vi "Oscillo2Data.vi"() -> ()   [LabVIEW 2023]
panel:
  out "standard error":string
  out "Extract path 2":path
  out "Current VI folder 2":path
  out "PNG file name 2":string
  out "Traces.txt 2":string
  out "Script.m path 2":path
  out "PDF file path 2":path
  out "Pixmap.bin path 2":path
  out "Traces.txt path 2":path
  in  "User interface":T1(tab)
  in  "User entries":enum32{""}(tab)
  in  "Customization":enum32{"Customization"}(tab)
  in  "Marker shape":string
  in  "Marker size":i32
  in  "Open PDF":bool
  in  "Open in MATLAB":bool
  in  "Colors":enum32{"Colors"}(tab)
  out "Corners":u32(colorbox)
  out "Traces":u32[](array[colorbox])
  in  "Size":enum32{"Size"}(tab)
  out "Depth":i32
  out "Width":i16
  out "Height":i16
  out "stdout":string
  in  "PNG file path":path
  out "Errors":string
  out "PNG picture":picture
  out "Current VI folder":path
  out "PNG file name":string
  out "Pixmap.bin path":path
  out "Traces.txt path":path
  out "Extract path":path
  out "Script.m path":path
  out "PDF file path":path
  out "Traces.txt":string
  in  "Arrays":enum32{"Arrays"}(tab)
  out "Pixels colors (uchar)":u32[](array[numeric])
  out "Pixels colors (CLUT)":u8[](array[numeric])
  out "Corners color (CLUT)":i32
  out "Traces colors (RGB)":u8[][](array[numeric])
  out "Traces colors (CLUT)":i32[](array[numeric])
  out "Traces colors string (RGB)":string[](array[string])
  out "Number of Traces":i32
  out "Script.m":string
  out "Colors error":errorcluster
  out "PNGFile error":errorcluster
  out "PixmapWrite error":errorcluster
  out "CallExtract error":errorcluster
  out "CallMATLAB out":errorcluster
  out "ScriptWrite error":errorcluster
  out "TracesRead error":errorcluster
  out "Paths error":errorcluster
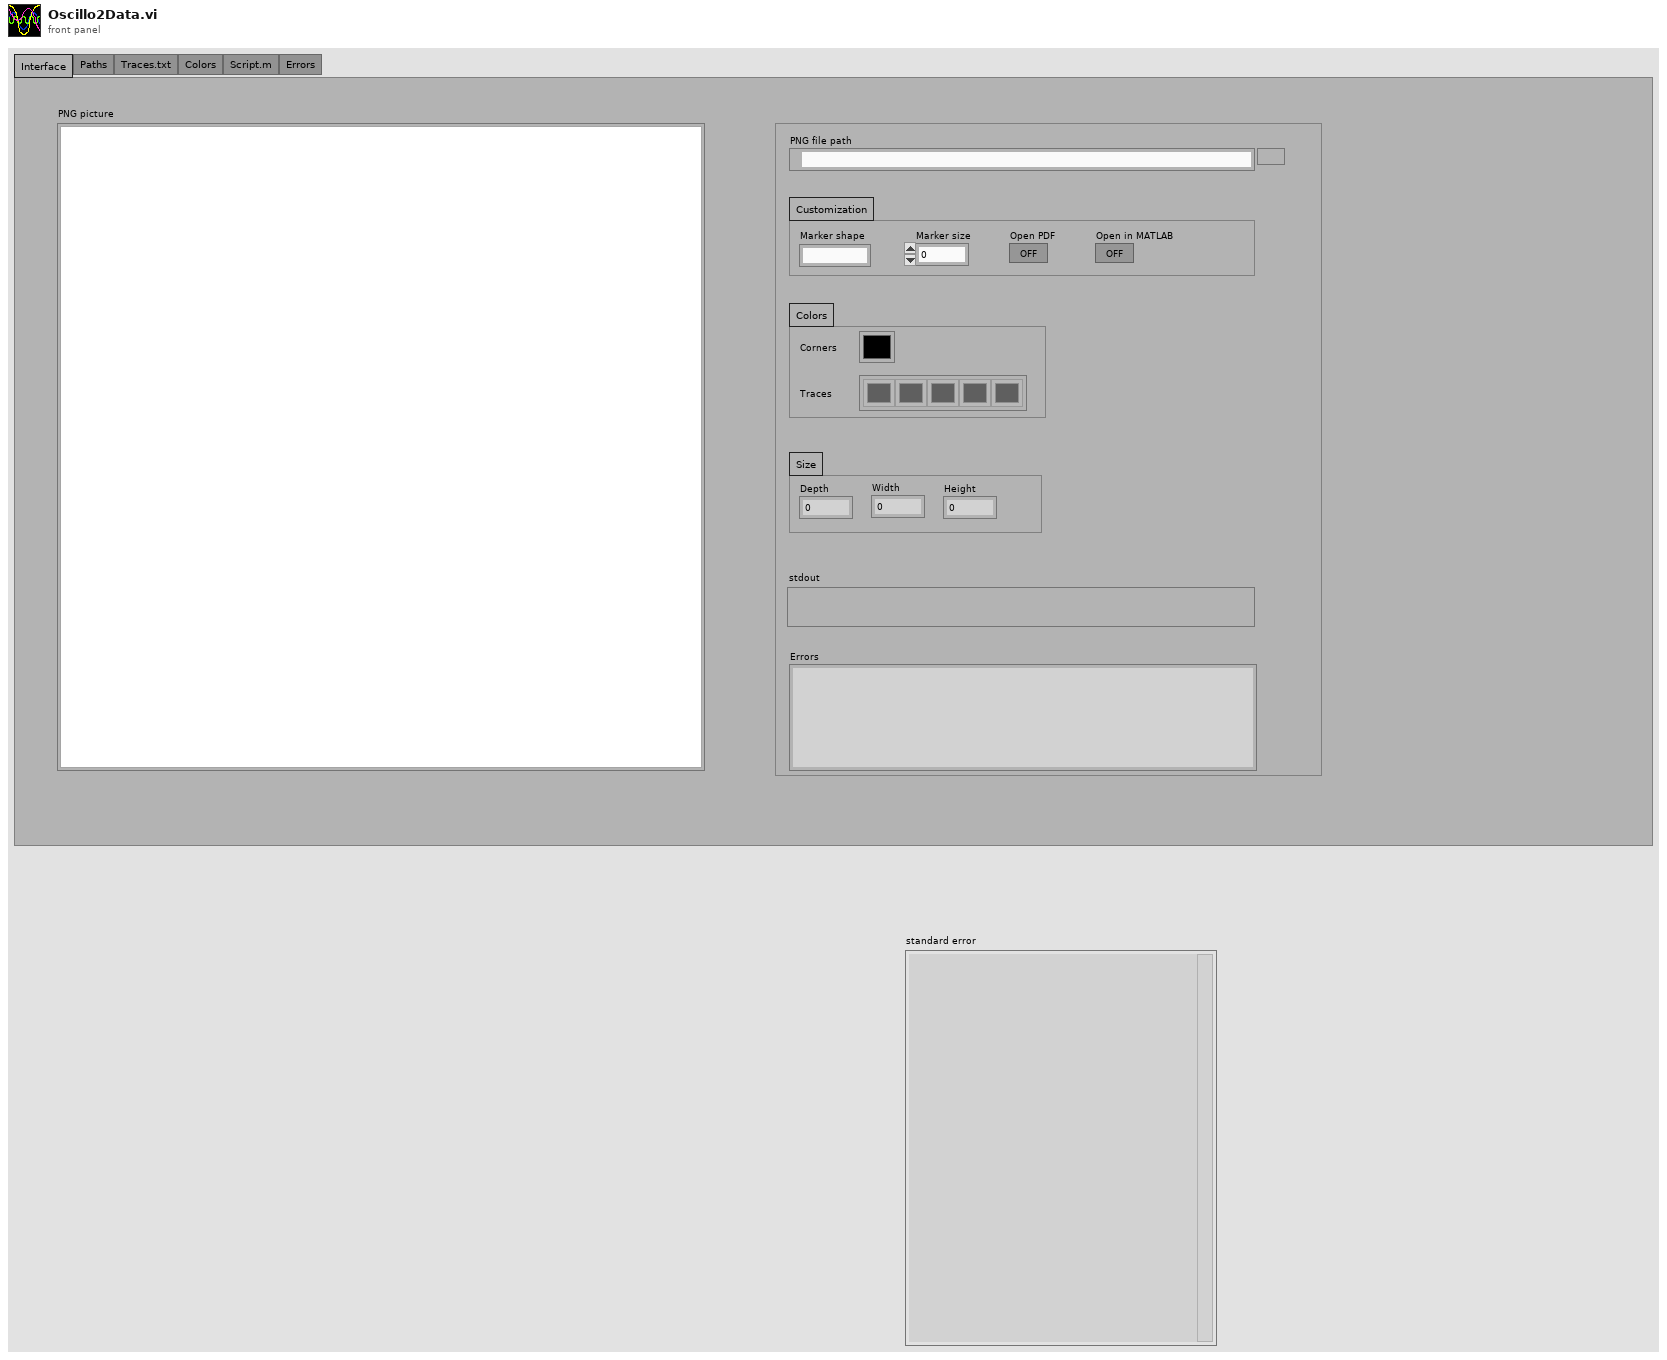
[diagram p1: front panel]
types:
  T1 = enum32{"Interface", "Paths", "Traces.txt", "Colors", "Script.m", "Errors"}
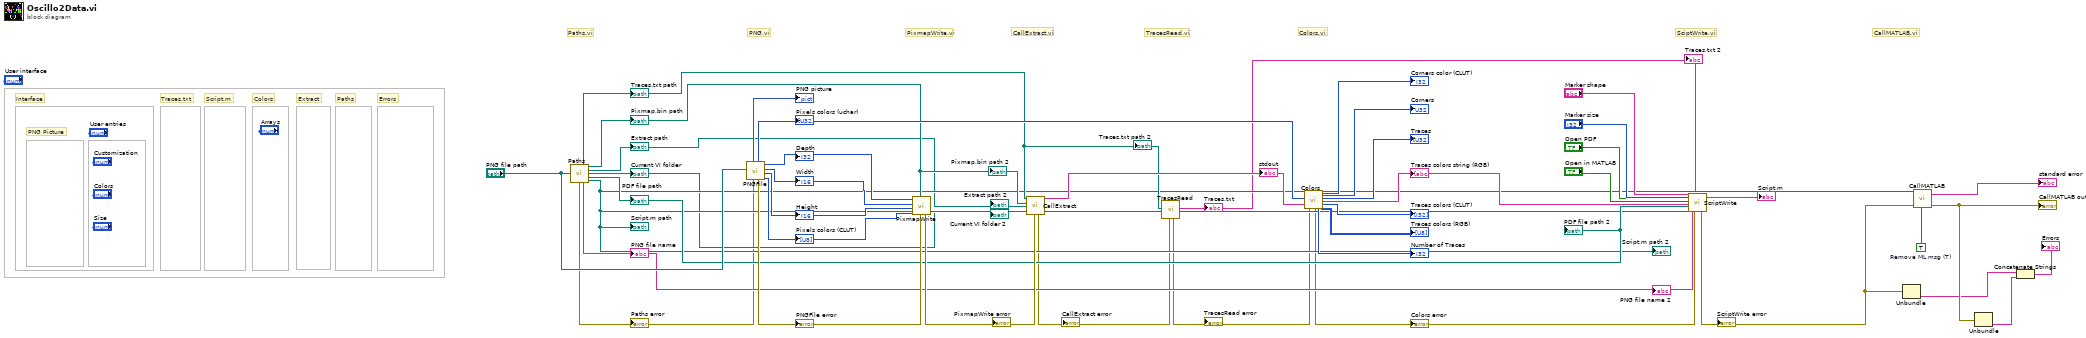
[diagram p0: block diagram]
diagram:
  w41 = TRUE  # Remove ML msg (T)
  # "CallMATLAB.vi"
  # "SciptWrite.vi"
  # "Colors.vi"
  # "TracesRead.vi"
  # "CallExtract.vi"
  # "PixmapWrite.vi"
  # "PNG.vi"
  # "Paths.vi"
  # "PNG Picture"
  # "Errors"
  # "Paths"
  # "Extract"
  # "Colors"
  # "Script.m"
  # "Traces.txt"
  # "Interface"
  n1 = call "Paths.vi"("PNG file path"="PNG file path") -> ("Traces.txt path"=w18:path, "Pixmap.bin path"=w17:path, "Extract path"=w12:path, "Current VI folder"=w13:path, "PDF file path"=w16:path, "Paths error"=w10:errorcluster, "PNG file name"=w11:string, "Script.m path"=w15:path)  [unwired: 7 in]
  "Traces.txt path" <- w18
  "Pixmap.bin path" <- w17
  "Extract path" <- w12
  "Current VI folder" <- w13
  "PDF file path" <- w16
  "Script.m path" <- w15
  "PNG file name" <- w11
  "Traces.txt path 2" <- w18
  "Pixmap.bin path 2" <- w17
  "PDF file path 2" <- w16
  "Script.m path 2" <- w15
  "PNG file name 2" <- w11
  "Current VI folder 2" <- w13
  "Extract path 2" <- w12
  "Paths error" <- w10
  n2 = call "PNGFile.vi"("Paths error"=w10, "PNG file path"="PNG file path") -> ("Pixels colors (CLUT)"=w37:u8[], "Height"=w38:i16, "Width"=w39:i16, "Depth"=w40:i32, "PNGFile error"=w36:errorcluster, "Pixels colors (uchar)"=w34:u32[], "PNG picture"=→"PNG picture":picture)  [unwired: 3 in]
  "Pixels colors (uchar)" <- w34
  "Depth" <- w40
  "Width" <- w39
  "Height" <- w38
  "Pixels colors (CLUT)" <- w37
  "PNGFile error" <- w36
  n3 = call "PixmapWrite.vi"("PNGFile error"=w36, "Pixmap.bin path"=w17, "Pixels colors (CLUT)"=w37, "Height"=w38, "Width"=w39, "Depth"=w40) -> ("Pixmap.bin error"=w35:errorcluster)  [unwired: 5 in]
  "PixmapWrite error" <- w35
  n4 = call "CallExtract.vi"("TracesRead error"=w35, "VI folder"=w13, "Extract path"=w12, "Pixmap.bin path"=w17, "Traces.txt path"=w18) -> ("stdout"=w33:string, "CallExtract error"=w5:errorcluster)  [unwired: 4 in, 1 out]
  "CallExtract error" <- w5
  "stdout" <- w33
  n5 = call "TracesRead.vi"("CallExtract error"=w5, "Traces.txt path"=w18) -> ("Traces.txt"=w14:string, "TracesRead error"=w9:errorcluster)  [unwired: 8 in]
  "TracesRead error" <- w9
  "Traces.txt" <- w14
  "Traces.txt 2" <- w14
  n6 = call "Colors.vi"("Pixels colors (uchar)"=w34, "stdout"=w33, "TracesRead error"=w9) -> ("Colors error"=w8:errorcluster, "Number of Traces"=→"Number of Traces":i32, "Corners color (CLUT)"=→"Corners color (CLUT)":i32, "Corners"=→"Corners":u32, "Traces"=→"Traces":u32[], "Traces colors string (RGB)"=w23:string[], "Traces colors (CLUT)"=→"Traces colors (CLUT)":i32[], "Traces colors (RGB)"=→"Traces colors (RGB)":u8[][])  [unwired: 9 in]
  "Traces colors string (RGB)" <- w23
  "Colors error" <- w8
  n7 = call "ScriptWrite.vi"("Marker shape"="Marker shape", "Marker size"="Marker size", "Open PDF"="Open PDF", "Open in MATLAB"="Open in MATLAB", "Traces colors string (RGB)"=w23, "PDF file path"=w16, "Script.m path"=w15, "Traces.txt"=w14, "PNG file name"=w11, "Colors error"=w8) -> ("ScriptWrite error"=w4:errorcluster, "Script.m"=→"Script.m":string)  [unwired: 16 in]
  "ScriptWrite error" <- w4
  n8 = Unbundle(w4) -> ("source"=w3:string)  [unwired: 2 out]
  n9 = call "CallMATLAB.vi"("Remove ML msg (T)"=w41, "error in (no error)"=w4, "matlab script path"=w15) -> ("error out"=w7:errorcluster, "standard error"=→"standard error":string)  [unwired: 3 in, 4 out]
  "CallMATLAB out" <- w7
  n10 = Unbundle(w7) -> ("source"=w2:string)  [unwired: 2 out]
  n11 = Concatenate Strings(w3, w2) -> (→"Errors":string)
